vi "Init.vi"(8 "error in (no error)":errorcluster, 11 "MassSpectrumExtractor in":refnum<class "MassSpectrumExtractor.lvclass">) -> (0 "error out":errorcluster, 3 "MassSpectrumExtractor out":refnum<class "MassSpectrumExtractor.lvclass">)   [LabVIEW 2014, in "MassSpectrumExtractor.lvclass"]
uses:
  MassSpectrumExtractor.lvclass
  Framework/Extractor/AbstractExtractor1D/AbstractExtractor1D.lvclass
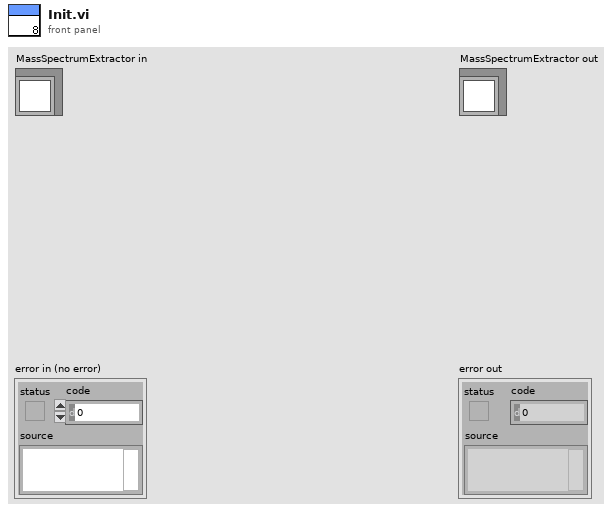
[diagram p1: front panel]
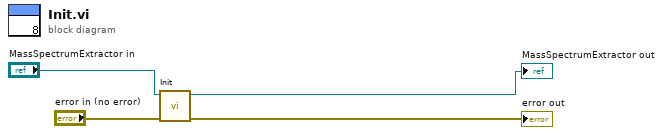
[diagram p0: block diagram]
diagram:
  n1 = call-parent "Init.vi"("error in (no error)"="error in (no error)", "AbstractExtractor in"="MassSpectrumExtractor in") -> ("error out"=→"error out":errorcluster, "AbstractExtractor out"=→"MassSpectrumExtractor out":refnum<class "MassSpectrumExtractor.lvclass">)  [unwired: 8 in]
